vi "Temperature monitor.vi"() -> ()   [LabVIEW 2011]
uses:
  <vilib>/Utility/error.llb/DialogType.ctl
  <vilib>/DAQmx/read.llb/DAQmx Read (Analog 2D DBL NChan NSamp).vi
  <vilib>/DAQmx/create/scale.llb/DAQmx Create Scale (Linear).vi
  <vilib>/DAQmx/create/channels.llb/DAQmx Create Channel (AI-Voltage-Basic).vi
  <vilib>/DAQmx/configure/timing.llb/DAQmx Timing (Sample Clock).vi
  <vilib>/DAQmx/miscellaneous.llb/DAQmx Fill In Error Info.vi
  <vilib>/Analysis/NI_AALBase.lvlib
panel:
  in  "stop":bool
  out "Waveform Chart":dbl[][](graph)
  in  "error in":errorcluster
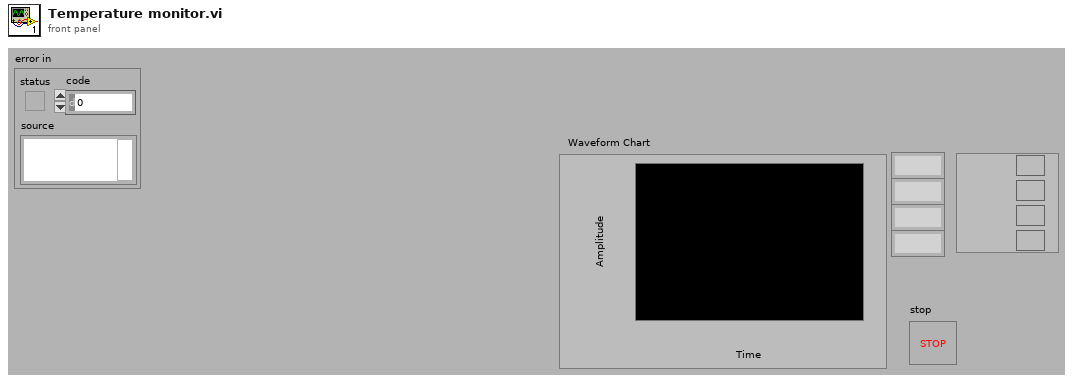
[diagram p1: front panel]
types:
  T1 = typedef "DialogType.ctl" = u16
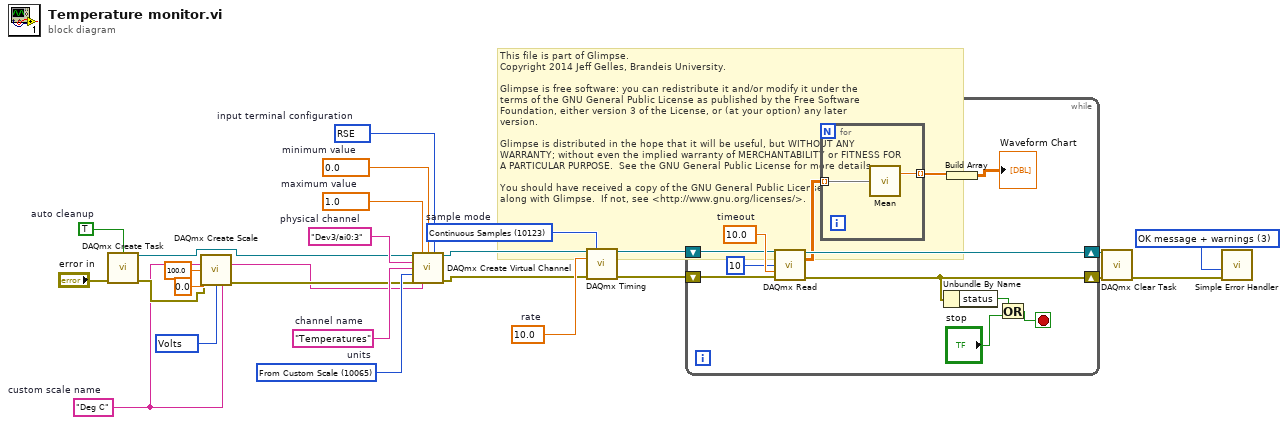
[diagram p0: block diagram]
diagram:
  w3 = 10348 items=["Volts"=10348, "Amps"=10342, "Deg F"=10144, "Deg C"=10143, "Deg R"=10145, "Kelvins"=10325, "Strain"=10299, "Ohms"=10384, "Hz"=10373, "Seconds"=10364, "Meters"=10219, "Inches"=10379, "Degrees"=10146, "Radians"=10273, "g"=10186, "m/s^2"=12470, "Pascals"=10081, "From TEDS"=12516] ("pre-scaled units")
  w13 = 10123 items=["Finite Samples"=10178, "Continuous Samples"=10123, "Hardware Timed Single Point"=12522]  # sample mode
  w14 = 10.0  # rate
  w15 = 10083 items=["default"=-1, "RSE"=10083, "NRSE"=10078, "Differential"=10106, "Pseudodifferential"=12529]  # input terminal configuration
  w16 = 10065 items=["Volts"=10348, "From Custom Scale"=10065]  # units
  w17 = "Temperatures"  # channel name
  w2 = "Deg C"  # custom scale name
  w18 = 0.0  # minimum value
  w19 = 1.0  # maximum value
  w20 = "Dev3/ai0:3"  # physical channel
  w21 = TRUE  # auto cleanup
  w26 = T1 3 items=["no dialog", "OK message", "continue or stop message", "OK message + warnings", "continue/stop + warnings"] ("type of dialog (OK msg:1)")
  # "This file is part of Glimpse. \nCopyright 2014 Jeff Gelles, Brandeis University.    \n\nGlimpse is free software: you can redistribute it and/or modify it under the \nterms of the GNU General Public License as published by the Free Software \nFoundation, either version 3 of the License, or (at your option) any later \nversion.\n\nGlimpse is distributed in the hope that it will be useful, but WITHOUT ANY \nWARRANTY; without even the implied warranty of MERCHANTABILITY or FITNESS FOR \nA PARTICULAR PURPOSE.  See the GNU General Public License for more details.\n\nYou should have received a copy of the GNU General Public License\nalong with Glimpse.  If not, see <http://www.gnu.org/licenses/>."
  n1 = call <vilib>:"DAQmx Create Task.vi"("auto cleanup"=w21, "error in"="error in") -> ("task out"=w8:refnum<k21>, "error out"=w5:errorcluster)  [unwired: 3 in, 9 out]
  n2 = call-poly <vilib>:"DAQmx Create Scale.vi"("name"=w2, "slope"=100.0, "y-intercept"=0.0, "error in"=w5, "pre-scaled units"=w3, "scaled units"=w2) -> ("scale out"=w1:tag, "error out"=w4:errorcluster)  [unwired: 8 out]
  n3 = call-poly <vilib>:"DAQmx Create Virtual Channel.vi"("task in"=w8, "maximum value"=w19, "minimum value"=w18, "input terminal configuration"=w15, "physical channels"=w20, "name to assign"=w17, "units"=w16, "error in"=w4, "custom scale name"=w1) -> ("task out"=w12:refnum<k21>, "error out"=w11:errorcluster)  [unwired: 5 out]
  n4 = call-poly <vilib>:"DAQmx Timing.vi"("task/channels in"=w12, "sample mode"=w13, "rate"=w14, "error in"=w11) -> ("task out"=w10:refnum<k21>, "error out"=w9:errorcluster)  [unwired: 3 in, 7 out]
  n5 = while {
    shift-right: [w31] -> w24
    shift-left: w9 -> [w35]
    shift-right: [w37] -> w25
    shift-left: w10 -> [w36]
    stop <- w33 stop-if-true
    w38 = 10.0  # timeout
    n6 = call-poly <vilib>:"DAQmx Read.vi"("task/channels in"=w36, "number of samples per channel"=10, "timeout"=w38, "error in"=w35) -> ("task out"=w37:refnum<k21>, "data"=w29:dbl[][], "error out"=w31:errorcluster)  [unwired: 9 out]
    n7 = for {
      tunnel: w29 -> [w40] mode=indexing
      tunnel: [w39] -> w28 mode=indexing
      n8 = call <vilib>:"Mean.vi"("X"=w40) -> ("mean"=w39:dbl)  [unwired: 1 out]
    }
    n9 = Unbundle By Name(w31) -> ("status"=w32:bool)
    n10 = Build Array(w28) -> (→"Waveform Chart":dbl[][])
    n11 = Or(x=w32, y="stop") -> (x .or. y?=w33:bool)
  }
  n12 = call <vilib>:"DAQmx Clear Task.vi"("task in"=w25, "error in"=w24) -> ("error out"=w23:errorcluster)  [unwired: 13 out]
  n13 = call <vilib>:"Simple Error Handler.vi"("type of dialog (OK msg:1)"=w26, "error in (no error)"=w23) -> ()  [unwired: 8 out]
